vi "PopulateControlsFromCSV2.vi"() -> ()   [LabVIEW 2019]
uses:
  <vilib>/Utility/file.llb/Read Delimited Spreadsheet (string).vi
panel:
  in  "Update":bool
  in  "Numeric1":dbl
  in  "Numeric2":dbl
  in  "Numeric3":dbl
  in  "Numeric4":dbl
  in  "Path":path=path "C:/Users/jbrus/Documents/GitHub/LabVIEW/3LabVIEWFeatures/PopulateControlsFromCSV/FileOutput.csv"
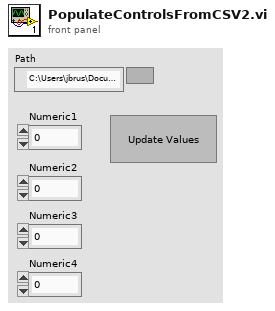
[diagram p1: front panel]
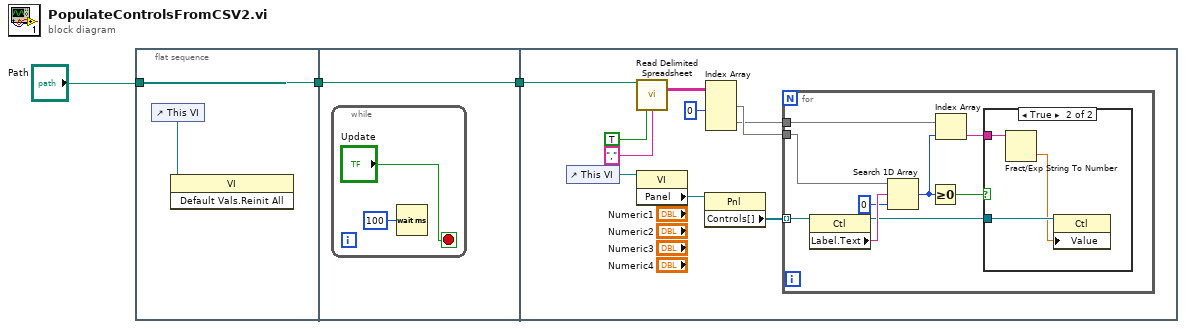
[diagram p0: block diagram]
diagram:
  n1 = flat-sequence {
    tunnel: [w4] -> w2
    tunnel: "Path" -> [w4]
    tunnel: w2 -> [w6]
    tunnel: [w6] -> w1
    tunnel: w1 -> [w9]
    frame #0 {
      n2 = control-ref of="This VI"() -> (w5:refnum<vi>)
      n3 = invoke class="VI" method="Default Vals.Reinit All"(reference=w5) -> ()  [unwired: 2 in, 3 out]
    }
    frame #1 {
      n4 = while {
        stop <- "Update" stop-if-true
        n5 = Wait (ms)(milliseconds to wait=u32 100) -> ()  [unwired: 1 out]
      }
    }
    frame #2 {
      n6 = control-ref of="This VI"() -> (w16:refnum<vi>)
      n7 = call-poly <vilib>:"Read Delimited Spreadsheet.vi"("file path (dialog if empty)"=w9, "transpose? (F)"=TRUE, "delimiter (\\t)"="," ("delimiter (\\t)")) -> ("all rows"=w13:string[][])  [unwired: 7 in, 5 out]
      n8 = property class="VI"(reference=w16) -> ("Panel"=w17:refnum<vi>)  [unwired: 1 in, 2 out]
      n9 = property class="Pnl"(reference=w17) -> ("Controls[]"=w18:refnum<vi>[])  [unwired: 1 in, 2 out]
      n10 = Index Array(array=w13, index (col) #1=0 ("disabled index (col)")) -> (element #1=w12:string[], element #2=w10:string[])  [unwired: 3 in]
      n11 = for {
        tunnel: w18 -> [w25] mode=indexing
        tunnel: w12 -> [w22]
        tunnel: w10 -> [w19]
        n12 = property class="Ctl"(reference=w25) -> (reference out=w24:refnum<vi>, "Label.Text"=w27:string)  [unwired: 1 in, 1 out]
        n13 = Search 1D Array(1D array=w22, element=w27, start index (0)=0) -> (index of element=w21:i32)
        n14 = Greater Or Equal To 0?(x=w21) -> (x >= 0?=w23:bool)
        n15 = Index Array(array=w19, index=w21) -> (element=w20:string)
        n16 = case shown="True" w23 {
          tunnel: w24 -> [_ w30]
          tunnel: w20 -> [_ w28]
          frame False {
          }
          frame True {
            n17 = Fract/Exp String To Number(string=w28) -> (number=w29:dbl)  [unwired: 3 in, 1 out]
            n18 = property class="Ctl"(reference=w30, "Value"=w29) -> ()  [unwired: 1 in, 2 out]
          }
        }
      }
    }
  }
